vi "Transfer Channel Count.vi"(8 "error in (no error)":errorcluster, 11 "Transfer Configuration in":T1 {"channel configurations"."buffer offset" format="%d bytes"}) -> (0 "error out":errorcluster, 2 "total channel count":u64, 3 "Transfer Configuration out":T1 {"channel configurations"."buffer offset" format="%d bytes"})   [LabVIEW 2017, in "DSF Core.lvlib"]
uses:
  DSF Core.lvlib
  Controls/DSF Engine Transfer Configuration.ctl
  Controls/DSF Byte Order.ctl
  Controls/DSF Engine Channel Configuration.ctl
  Controls/DSF Data Type.ctl
  Controls/DSF Settings Info.ctl
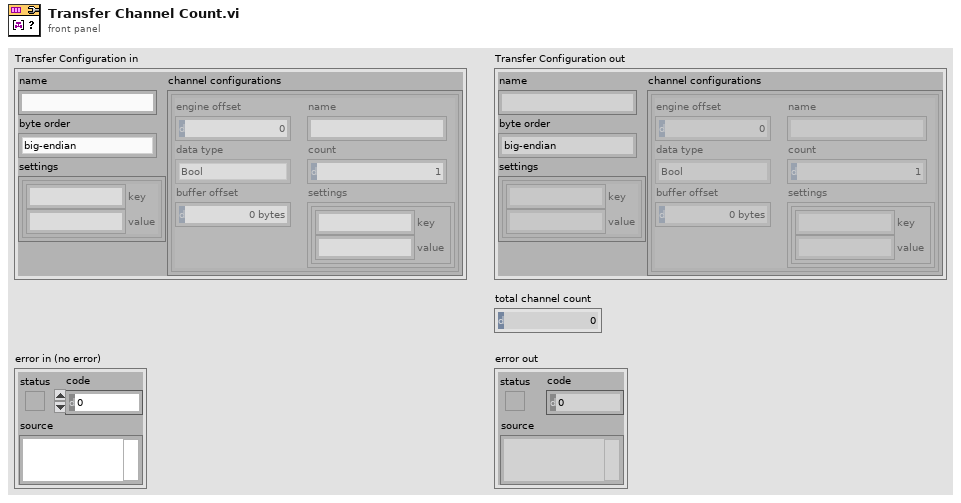
[diagram p1: front panel]
types:
  T1 = typedef "DSF Core.lvlib/DSF Engine Transfer Configuration.ctl" = cluster{"name":string, "byte order":T2, "channel configurations":T3[], "settings":T5}
  T2 = typedef "DSF Core.lvlib/DSF Byte Order.ctl" = enum8{"big-endian", "little-endian"}
  T3 = typedef "DSF Core.lvlib/DSF Engine Channel Configuration.ctl" = cluster{"engine offset":u64, "name":string, "data type":T4, "count":u64, "buffer offset":u64, "settings":T5}
  T4 = typedef "DSF Core.lvlib/DSF Data Type.ctl" = enum8{"Bool", "SGL", "DBL", "I8", "I16", "I32", "I64", "U8", "U16", "U32", "U64"}
  T5 = typedef "DSF Core.lvlib/DSF Settings Info.ctl" = cluster{"key":string, "value":string}[]
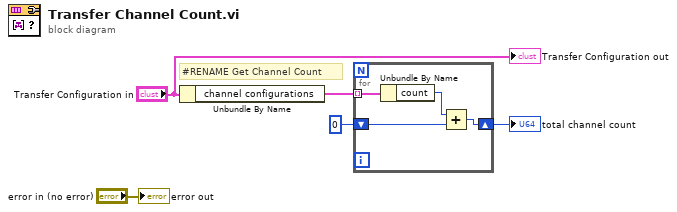
[diagram p0: block diagram]
diagram:
  # "#RENAME Get Channel Count"
  n1 = Unbundle By Name("Transfer Configuration in") -> ("channel configurations"=w1:T3[])
  n2 = for {
    tunnel: w1 -> [w9] mode=indexing
    shift-right: [w6] -> w3
    shift-left: u64 0 -> [w8]
    n3 = Unbundle By Name(w9) -> ("count"=w7:u64)
    n4 = Add(x=w7, y=w8) -> (x+y=w6:u64)
  }
  "total channel count" <- w3
  "error out" <- "error in (no error)"
  "Transfer Configuration out" <- "Transfer Configuration in"
